vi "Get Certificate Details.vi"(8 "error in (no error)":errorcluster, 10 "Certificate ID":string, 11 "IoT Session in":refnum<class "IoT Session.lvclass">) -> (0 "error out":errorcluster, 2 "Certificate Details":T1 {"Transfer Data"."Transfer Date" format="%#_12g"; "Transfer Data"."Reject Date" format="%#_12g"; "Transfer Data"."Accept Date" format="%#_12g"; "Last Modified Date" format="%#_12g"; "Creation Date" format="%#_12g"}, 3 "IoT Session out":refnum<class "IoT Session.lvclass">)   [LabVIEW 2015, in "NI_AWS_IoT.lvlib" / "IoT Session.lvclass"]
uses:
  IoT Session.lvclass
  Certificate Details.ctl
  Certificate Status.ctl
  Transfer Data.ctl
  Core/HTTP Request/Request Options.ctl
  Core/HTTP Request/Name Value Pair.ctl
  Core/HTTP Request/Region handling.ctl
  Core/HTTP Request/URL formatting.ctl
  Core/HTTP Request/HTTP Request.lvclass
  JSON Parsing/NI_JSON Parsing.lvlib
  NI_AWS_IoT.lvlib
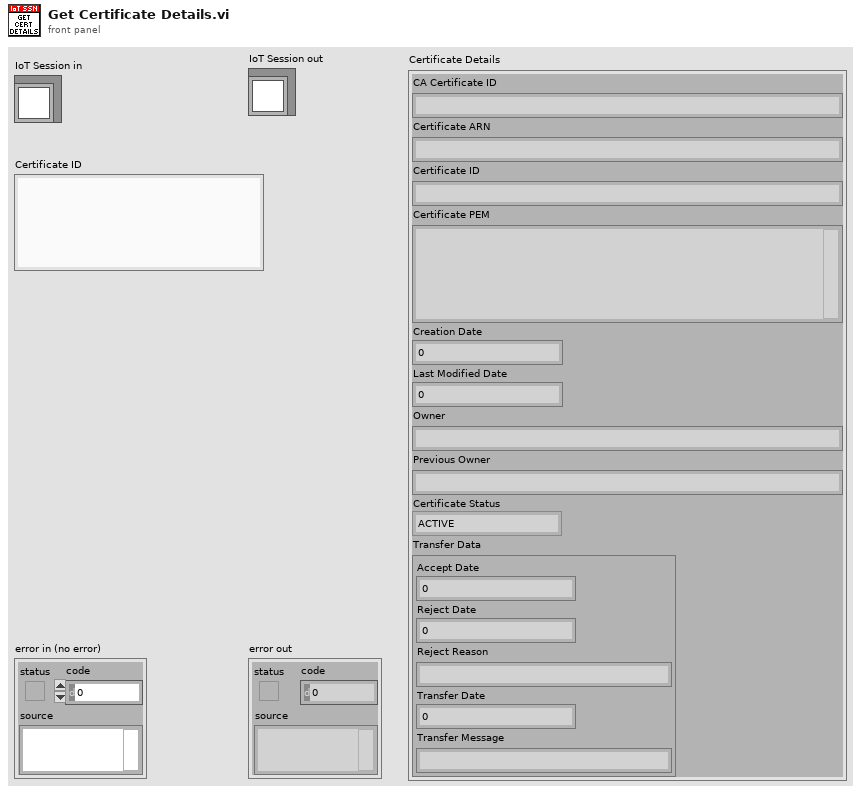
[diagram p1: front panel]
types:
  T1 = typedef "NI_AWS_IoT.lvlib/Certificate Details.ctl" = cluster{"CA Certificate ID":string, "Certificate ARN":string, "Certificate ID":string, "Certificate PEM":string, "Creation Date":dbl, "Last Modified Date":dbl, "Owner":string, "Previous Owner":string, "Certificate Status":T2, "Transfer Data":T3}
  T2 = typedef "NI_AWS_IoT.lvlib/Certificate Status.ctl" = enum16{"ACTIVE", "INACTIVE", "REVOKED", "PENDING_TRANSFER", "REGISTER_INACTIVE", "PENDING_ACTIVATION"}
  T3 = typedef "NI_AWS_IoT.lvlib/Transfer Data.ctl" = cluster{"Accept Date":dbl, "Reject Date":dbl, "Reject Reason":string, "Transfer Date":dbl, "Transfer Message":string}
  T4 = typedef "NI_AWS_Core.lvlib/HTTP Request.lvclass/Name Value Pair.ctl" = cluster{"name":string, "value":string}
  T5 = typedef "NI_AWS_Core.lvlib/HTTP Request.lvclass/Request Options.ctl" = cluster{"request headers":T4[], "request parameters":T4[], "request body":string, "region handling":T6, "URL formatting":T7}
  T6 = typedef "NI_AWS_Core.lvlib/HTTP Request.lvclass/Region handling.ctl" = enum16{"use region everywhere", "use region (authentication only)", "use region (URL only)", "ignore region everwhere"}
  T7 = typedef "NI_AWS_Core.lvlib/HTTP Request.lvclass/URL formatting.ctl" = enum16{"region-", "region."}
  T8 = typedef "NI_AWS_Core.lvlib/HTTP Request.lvclass/Response.ctl" = cluster{"Headers":string, "Body":string}
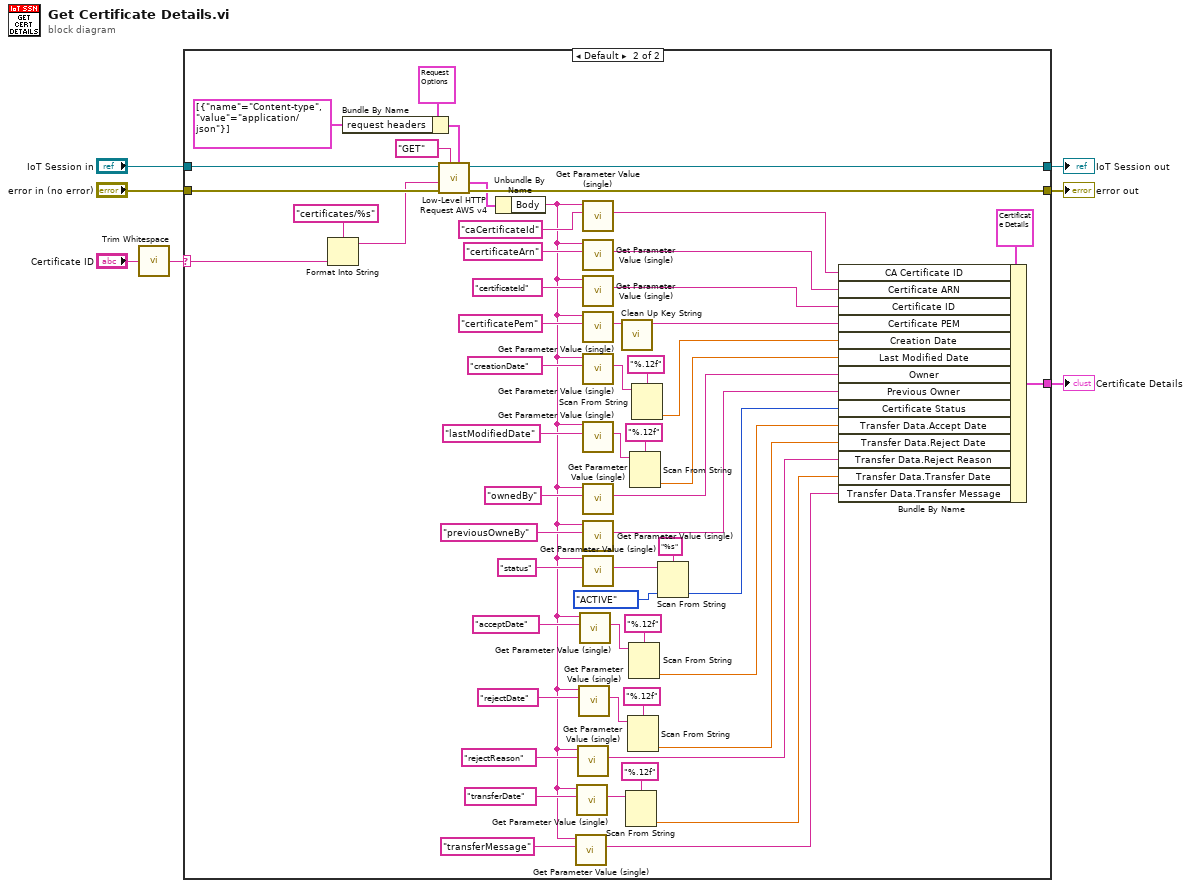
[diagram p0: block diagram]
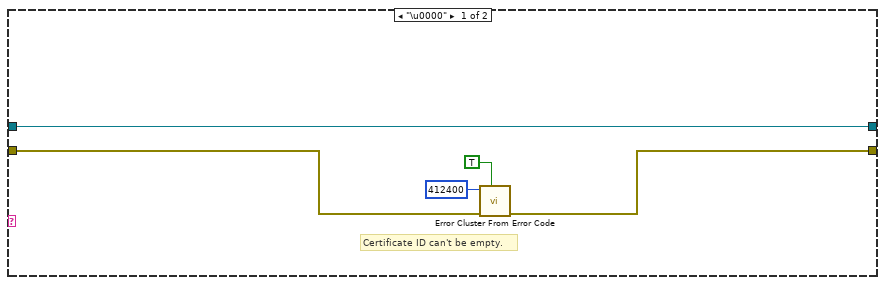
[diagram p2: hidden frame]
diagram:
  n1 = call <vilib>:"Trim Whitespace.vi"("string"="Certificate ID") -> ("trimmed string"=w1:string)  [unwired: 1 in]
  n2 = case shown="Default" w1 {
    selector: w1 -> [_ w53]
    tunnel: "error in (no error)" -> [w9 w69]
    tunnel: [w8 w68] -> w6
    tunnel: [w12 w67] -> w5
    tunnel: "IoT Session in" -> [w12 w66]
    tunnel: [_ w30] -> w2
    frame "\u0000" {
      # "Certificate ID can't be empty."
      n3 = call <vilib>:"Error Cluster From Error Code.vi"("show call chain? (False)"=TRUE, "error in (no error)"=w9, "error code (0)"=412400) -> ("error out"=w8:errorcluster)  [unwired: 6 in]
    }
    frame Default {
      n4 = Format Into String(format string="certificates/%s", w53) -> (resulting string=w52:string)  [unwired: 2 in, 1 out]
      n5 = Bundle By Name(cluster=T5 {"request headers"=[], "request parameters"=[], "request body"="", "region handling"=enum."use region everywhere", "URL formatting"=enum."region."} ("Request Options"), "request headers"=T4[] [{"name"="Content-type", "value"="application/json"}]) -> (w63:T5)
      n6 = call "Low-Level HTTP Request AWS v4.vi"("Request Options"=w63, "HTTP-Verb"="GET", "error in (no error)"=w69, "URL Suffix"=w52, "AWS Core in"=w66) -> ("error out"=w68:errorcluster, "Response"=w61:T8, "AWS Core out"=w67:refnum<class "IoT Session.lvclass">)  [unwired: 3 in, 1 out]
      n7 = Unbundle By Name(w61) -> ("Body"=w13:string)
      n8 = call "Get Parameter Value (single).vi"("Parameter Name"="transferMessage", "JSON"=w13) -> ("Parameter Value"=w14:string)  [unwired: 6 in, 3 out]
      n9 = call "Get Parameter Value (single).vi"("Parameter Name"="transferDate", "JSON"=w13) -> ("Parameter Value"=w19:string)  [unwired: 6 in, 3 out]
      n10 = call "Get Parameter Value (single).vi"("Parameter Name"="rejectReason", "JSON"=w13) -> ("Parameter Value"=w20:string)  [unwired: 6 in, 3 out]
      n11 = call "Get Parameter Value (single).vi"("Parameter Name"="rejectDate", "JSON"=w13) -> ("Parameter Value"=w23:string)  [unwired: 6 in, 3 out]
      n12 = call "Get Parameter Value (single).vi"("Parameter Name"="acceptDate", "JSON"=w13) -> ("Parameter Value"=w29:string)  [unwired: 6 in, 3 out]
      n13 = call "Get Parameter Value (single).vi"("Parameter Name"="caCertificateId", "JSON"=w13) -> ("Parameter Value"=w50:string)  [unwired: 6 in, 3 out]
      n14 = call "Get Parameter Value (single).vi"("Parameter Name"="certificateArn", "JSON"=w13) -> ("Parameter Value"=w49:string)  [unwired: 6 in, 3 out]
      n15 = call "Get Parameter Value (single).vi"("Parameter Name"="certificateId", "JSON"=w13) -> ("Parameter Value"=w48:string)  [unwired: 6 in, 3 out]
      n16 = call "Get Parameter Value (single).vi"("Parameter Name"="certificatePem", "JSON"=w13) -> ("Parameter Value"=w55:string)  [unwired: 6 in, 3 out]
      n17 = call "Get Parameter Value (single).vi"("Parameter Name"="creationDate", "JSON"=w13) -> ("Parameter Value"=w45:string)  [unwired: 6 in, 3 out]
      n18 = call "Get Parameter Value (single).vi"("Parameter Name"="lastModifiedDate", "JSON"=w13) -> ("Parameter Value"=w43:string)  [unwired: 6 in, 3 out]
      n19 = call "Get Parameter Value (single).vi"("Parameter Name"="ownedBy", "JSON"=w13) -> ("Parameter Value"=w38:string)  [unwired: 6 in, 3 out]
      n20 = call "Get Parameter Value (single).vi"("Parameter Name"="previousOwneBy", "JSON"=w13) -> ("Parameter Value"=w36:string)  [unwired: 6 in, 3 out]
      n21 = call "Get Parameter Value (single).vi"("Parameter Name"="status", "JSON"=w13) -> ("Parameter Value"=w34:string)  [unwired: 6 in, 3 out]
      n22 = call "Clean Up Key String.vi"("Key"=w55) -> ("Cleaned Up Key"=w47:string)  [unwired: 10 in]
      n23 = Scan From String(format string="%.12f", input string=w19) -> (output 1=w16:dbl)  [unwired: 3 in, 3 out]
      n24 = Scan From String(format string="%.12f", input string=w23) -> (output 1=w22:dbl)  [unwired: 3 in, 3 out]
      n25 = Scan From String(format string="%.12f", input string=w29) -> (output 1=w26:dbl)  [unwired: 3 in, 3 out]
      n26 = Scan From String(format string="%.12f", input string=w43) -> (output 1=w40:dbl)  [unwired: 3 in, 3 out]
      n27 = Scan From String(format string="%.12f", input string=w45) -> (output 1=w44:dbl)  [unwired: 3 in, 3 out]
      n28 = Scan From String(format string="%s", input string=w34, default 1=Certificate_Status."ACTIVE" ("Certificate Status")) -> (output 1=w31:T2)  [unwired: 2 in, 3 out]
      n29 = Bundle By Name(cluster=T1 {"CA Certificate ID"="", "Certificate ARN"="", "Certificate ID"="", "Certificate PEM"="", "Creation Date"=0.0, "Last Modified Date"=0.0, "Owner"="", "Previous Owner"="", "Certificate Status"=enum."ACTIVE", "Transfer Data"={"Accept Date"=0.0, "Reject Date"=0.0, "Reject Reason"="", "Transfer Date"=0.0, "Transfer Message"=""}} ("Certificate Details"), "CA Certificate ID"=w50, "Certificate ARN"=w49, "Certificate ID"=w48, "Certificate PEM"=w47, "Creation Date"=w44, "Last Modified Date"=w40, "Owner"=w38, "Previous Owner"=w36, "Certificate Status"=w31, "Transfer Data.Accept Date"=w26, "Transfer Data.Reject Date"=w22, "Transfer Data.Reject Reason"=w20, "Transfer Data.Transfer Date"=w16, "Transfer Data.Transfer Message"=w14) -> (w30:T1)
    }
  }
  "error out" <- w6
  "IoT Session out" <- w5
  "Certificate Details" <- w2
